vi "PDCConvertResolution.vi"(10 "ResValue":u16, 11 "ResStrings":string[](array[string])) -> (2 "Height":u32, 3 "Width":u32)   [LabVIEW 2015]
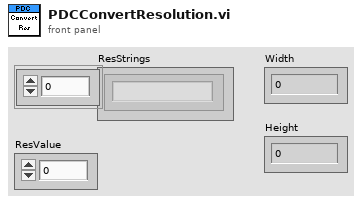
[diagram p1: front panel]
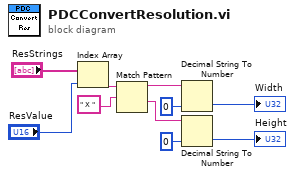
[diagram p0: block diagram]
diagram:
  n1 = Index Array(array="ResStrings", index="ResValue") -> (element=w6:string)
  n2 = Match Pattern(string=w6, regular expression=" X ") -> (before substring=w3:string, after substring=w1:string)  [unwired: 3 out]
  n3 = Decimal String To Number(string=w3, default (0L)=u32 0 ("デフォルト (0 I32)")) -> (number=→"Width":u32)  [unwired: 2 out]
  n4 = Decimal String To Number(string=w1, default (0L)=u32 0 ("デフォルト (0 I32)")) -> (number=→"Height":u32)  [unwired: 2 out]
